vi "Resolve-sender.vi"(8 "error in (no error)":errorcluster, 11 "Message":refnum<class "Message.lvclass">) -> (0 "error out":errorcluster, 1 "Sender ID":i32, 2 "Sender type":T1, 3 "Message dup":refnum<class "Message.lvclass">)   [LabVIEW 2013, in "Client.lvlib" / "Client.lvclass"]
uses:
  Client.lvclass
  Messages/Sources/Message.lvclass
  Supported-modules.ctl
  Messages/Sources/Message.lvclass/Message.ctl
  Custom-errors.ctl
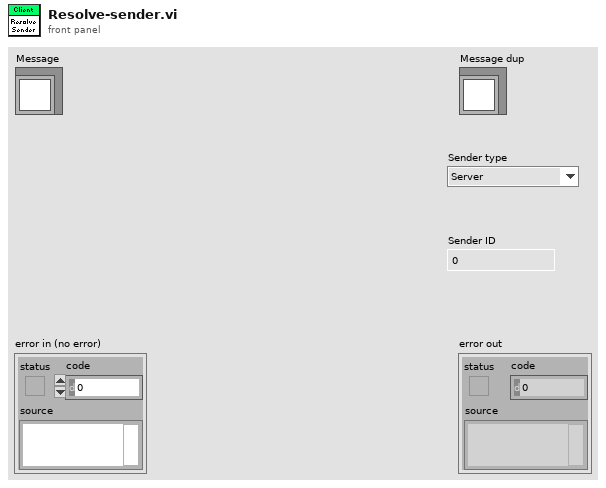
[diagram p1: front panel]
types:
  T1 = typedef "Client.lvlib/Client.lvclass/Supported-modules.ctl" = enum16{"Server", "All", "BeamControl", "PowderDeposition", "StrategyParser", "CameraVision", "MaterialCharacterization", "StatusMonitor", "SLMSimulation", "LaserCharacterization"}
  T2 = typedef "Client.lvlib/Client.lvclass/Custom-errors.ctl" = enum16{"No error", "Command not recognized", "Invalid input", "Timeout", "Not implemented", "Unsupported message", "Unsupported client", "Unsupported action"}
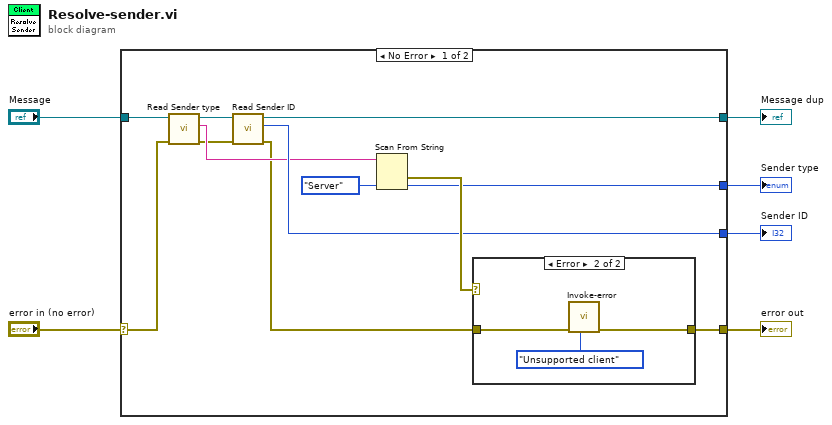
[diagram p0: block diagram]
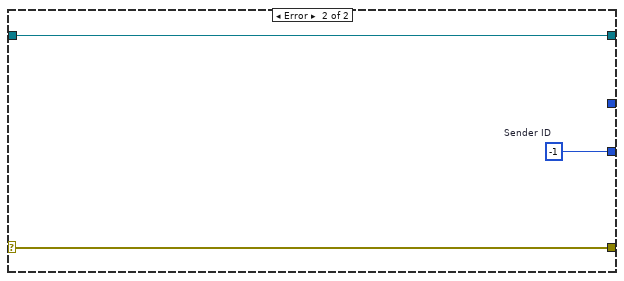
[diagram p3: hidden frame]
diagram:
  n1 = case shown="No Error" "error in (no error)" {
    selector: "error in (no error)" -> [w10 w25]
    tunnel: [w7 w25] -> w5
    tunnel: "Message" -> [w18 w24]
    tunnel: [w14 w24] -> w3
    tunnel: [w11 _] -> w2
    tunnel: [w13 w23] -> w1
    frame No Error {
      n2 = call "Read Sender type.vi"("error in (no error)"=w10, "Message in"=w18) -> ("error out"=w9:errorcluster, "Sender type"=w12:string, "Message out"=w17:refnum<class "Message.lvclass">)  [unwired: 7 in]
      n3 = call "Read Sender ID.vi"("error in (no error)"=w9, "Message in"=w17) -> ("error out"=w8:errorcluster, "Sender ID"=w13:i32, "Message out"=w14:refnum<class "Message.lvclass">)  [unwired: 7 in]
      n4 = Scan From String(input string=w12, default 1=Supported-modules."Server" ("Module type")) -> (error out=w15:errorcluster, output 1=w11:T1)  [unwired: 3 in, 2 out]
      n5 = case shown="Error" w15 {
        tunnel: w8 -> [w19 w22]
        tunnel: [w19 w21] -> w7
        frame No Error {
        }
        frame Error {
          n6 = call "Invoke-error.vi"("Error"=Custom-errors."Unsupported client", "error in (no error)"=w22) -> ("error out"=w21:errorcluster)  [unwired: 9 in]
        }
      }
    }
    frame Error {
      w23 = -1  # Sender ID
    }
  }
  "error out" <- w5
  "Message dup" <- w3
  "Sender type" <- w2
  "Sender ID" <- w1
